vi "template-state-machine-cDAQ-AO.vi"() -> ()   [LabVIEW 2024]
uses:
  state-enum.ctl
  utils-sub-vi/csv-file-logging-util/filepath-selection.ctl
  utils-sub-vi/csv-file-logging-util/datalogging-options.ctl
  cDAQ-options.ctl
  sensor-options.ctl
  <vilib>/DAQmx/write.llb/DAQmx Write (Analog DBL 1Chan 1Samp).vi
  <vilib>/DAQmx/create/channels.llb/DAQmx Create Channel (AO-Voltage-Basic).vi
  <vilib>/DAQmx/miscellaneous.llb/DAQmx Fill In Error Info.vi
panel:
  out "Log File Open":bool
  in  "Tab Control":enum32{"Data", "Settings"}(tab)
  out "Vout":dbl
  in  "Pressure (Bar)":dbl(slide) min=0.0 max=3.0 scale=0.0..3.0
  out "Logged CSV out":string
  in  "Datalogging options":T1={"data-precision"=3, "Include Date"=FALSE, "Include Timestamp"=TRUE, "Include Milliseconds"=FALSE, "sample-rate (Hz)"=4.0, "Logging Active"=FALSE}
  in  "Log Filepath Selection":T2={"Log Filepath Source"=enum."Application Relative (Auto)", "Log File Path (Manual)"=path "C:/Users/dheard/Documents/0002-labview-projects/labview-template-state-machine/data", "Log File Folder Name"="data", "log file name"="log", "Include Date in Filename"=TRUE, "Include Time in Filename"=TRUE}
  in  "Serial Port Options":T3={"AO Channel"="cDAQ3Mod1/ao0", "AI Channel"="", "Simulate Hardware"=FALSE}
  in  "Sensor Options":T4={"Display Units"="PSI", "Zero Offset"=0.0, "Sensor Min"=0.0, "Sensor Max"=5.0, "Signal Min"=0.0, "Signal Max"=3.0, "Conversion Factor"=0.0}
  in  "save-settings":bool
  in  "load-settings":bool
  in  "Settings file":path
  out "Sample Rate (Hz)":dbl format="%-#3.3f"
  in  "Debug Mode":bool
  out "Loop Time (mS)":u32
  out "State:":T5
  out "error IO":errorcluster
  in  "stop":bool
  in  "start":bool
  in  "Exit":bool
  # "Template Logger"
  # "Conversion Factor to\nCalculate User Units from Sensor Units"
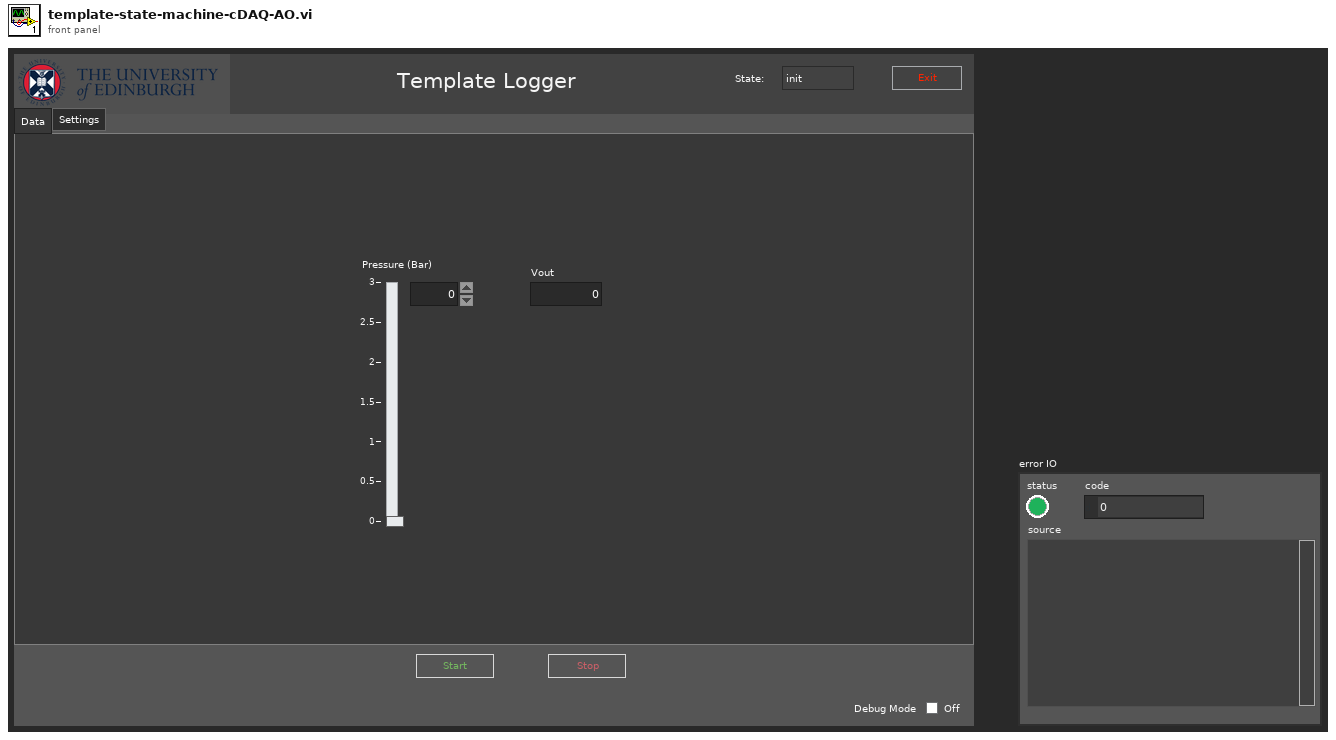
[diagram p1: front panel]
types:
  T1 = typedef "datalogging-options.ctl" = cluster{"data-precision":i32, "Include Date":bool, "Include Timestamp":bool, "Include Milliseconds":bool, "sample-rate (Hz)":dbl, "Logging Active":bool}
  T2 = typedef "filepath-selection.ctl" = cluster{"Log Filepath Source":enum16{"Application Relative (Auto)", "VI Relative (Auto)", "Complete Path (Manual)"}, "Log File Path (Manual)":path, "Log File Folder Name":string, "log file name":string, "Include Date in Filename":bool, "Include Time in Filename":bool}
  T3 = typedef "cDAQ-options.ctl" = cluster{"AO Channel":tag, "AI Channel":tag, "Simulate Hardware":bool}
  T4 = typedef "sensor-options.ctl" = cluster{"Display Units":string, "Zero Offset":dbl, "Sensor Min":dbl, "Sensor Max":dbl, "Signal Min":dbl, "Signal Max":dbl, "Conversion Factor":dbl}
  T5 = typedef "state-enum.ctl" = enum16{"init", "recall-settings", "save-settings", "wait", "start", "pre-run", "run", "stop", "shutdown", "exit"}
  T6 = enum8{"Enabled", "Disabled", "Disabled and Grayed Out"}
  T7 = enum16{"open", "replace", "create", "open or create", "replace or create", "replace or create with confirmation"}
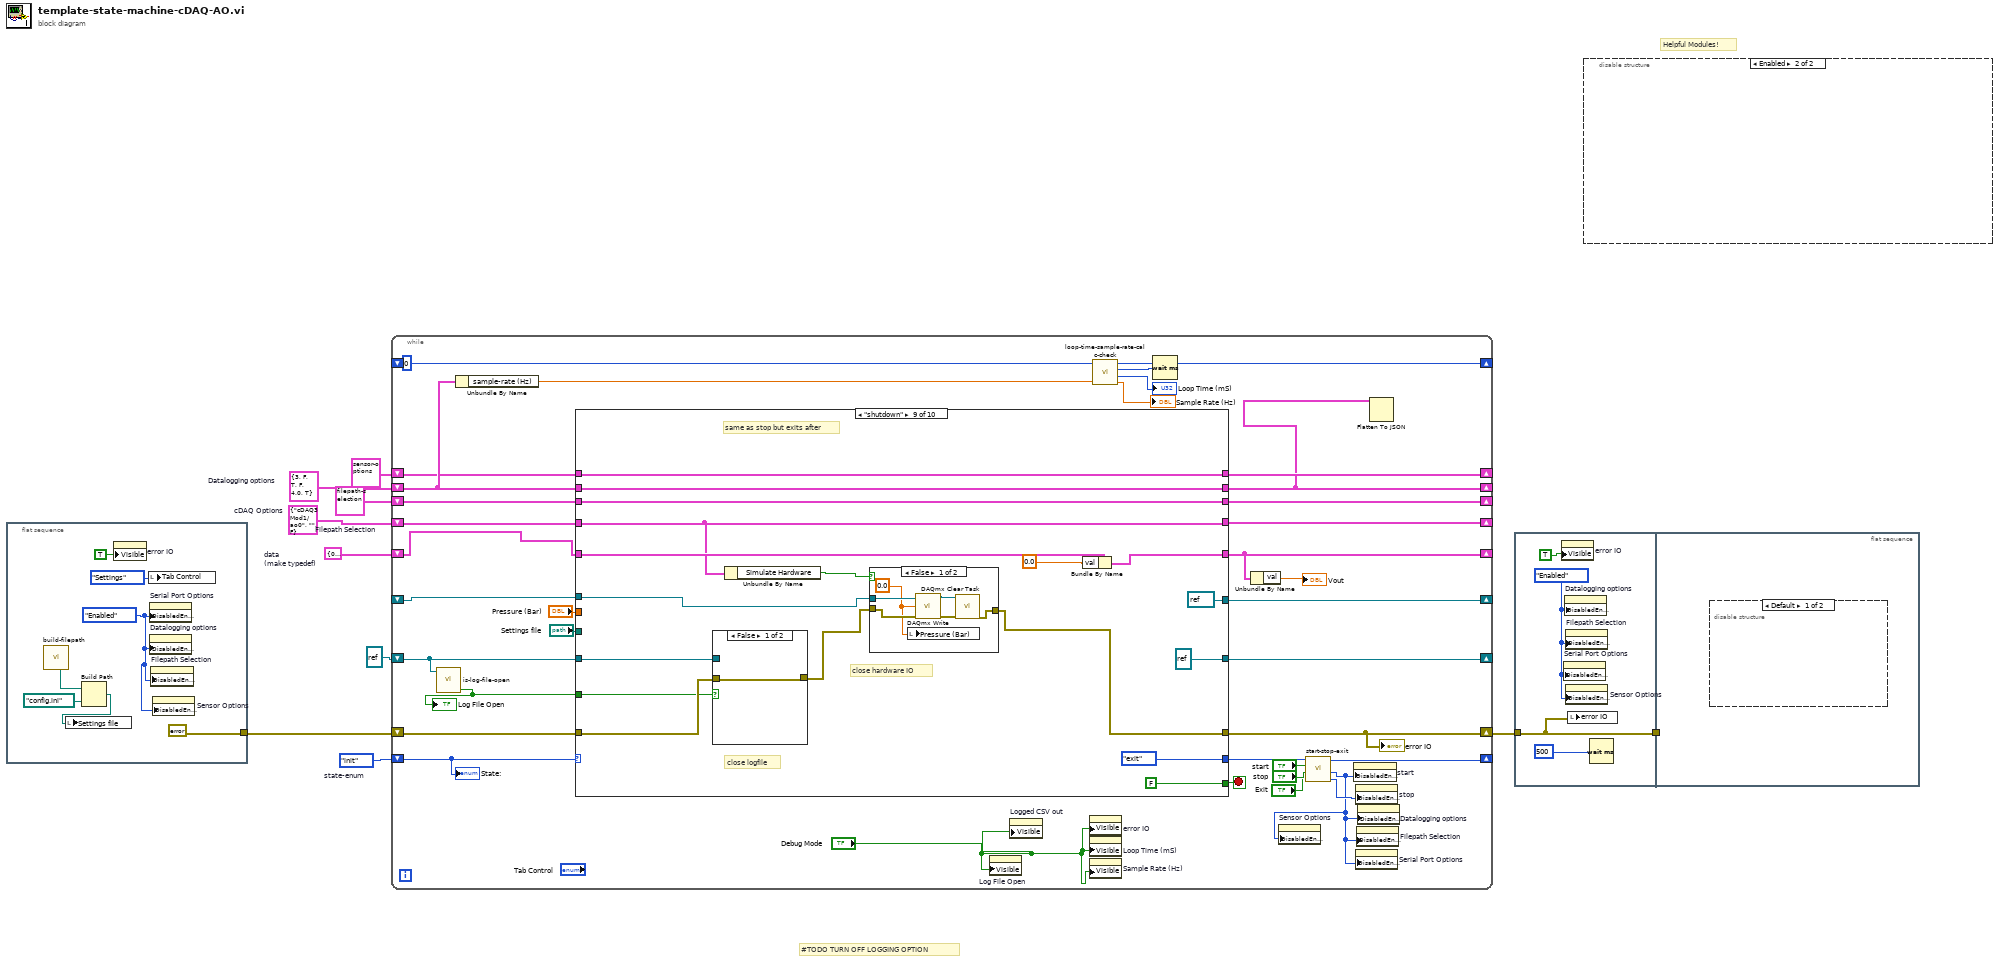
[diagram p0: block diagram]
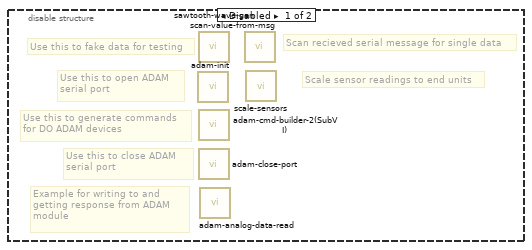
[diagram p2: hidden frame]
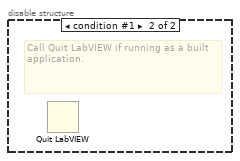
[diagram p3: hidden frame]
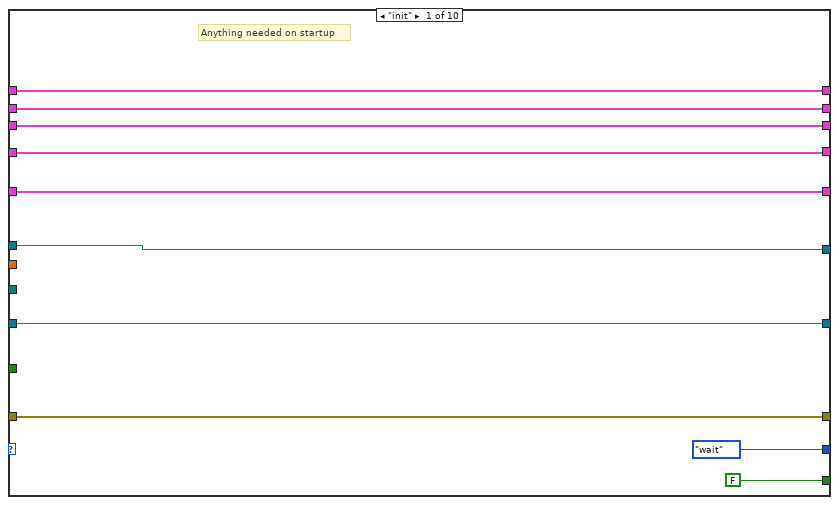
[diagram p4: hidden frame]
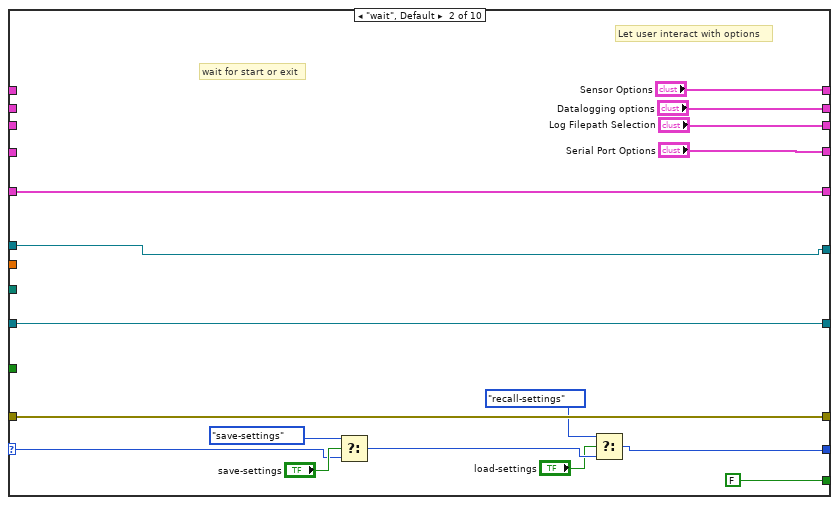
[diagram p5: hidden frame]
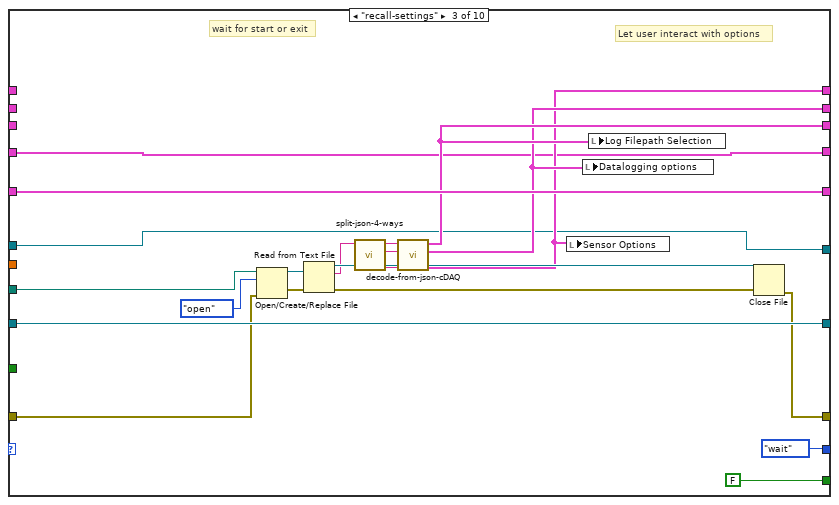
[diagram p6: hidden frame]
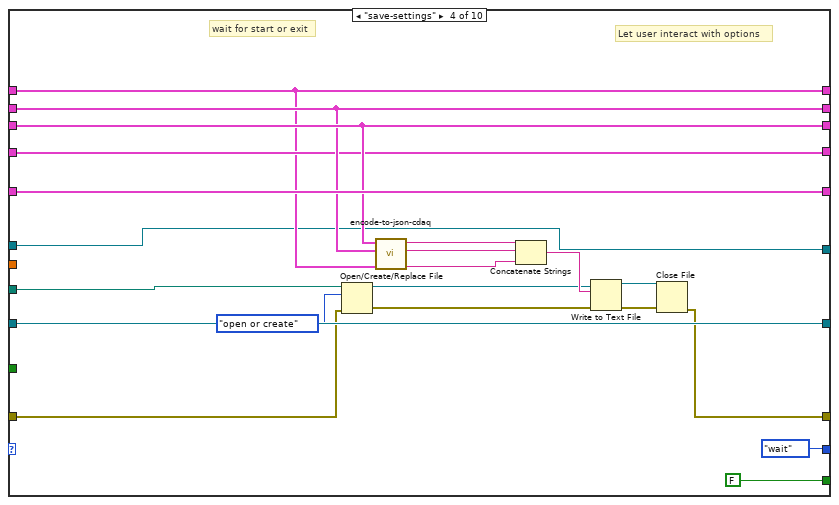
[diagram p7: hidden frame]
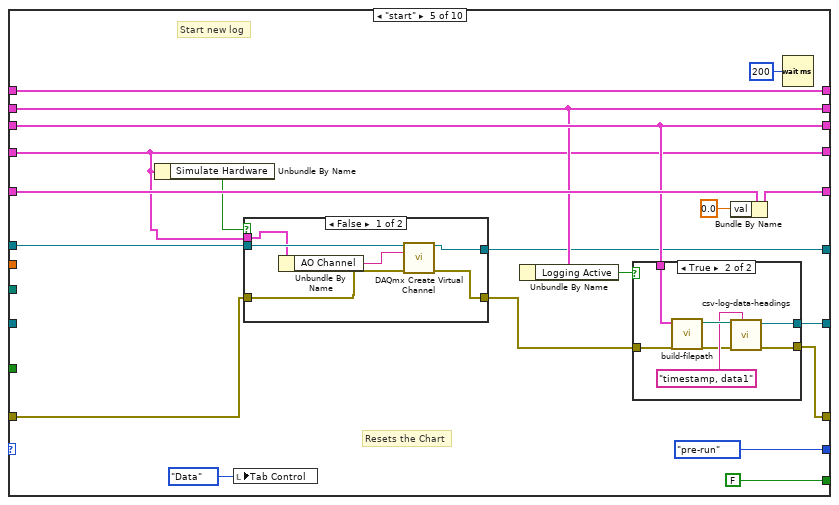
[diagram p8: hidden frame]
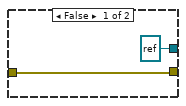
[diagram p10: hidden frame]
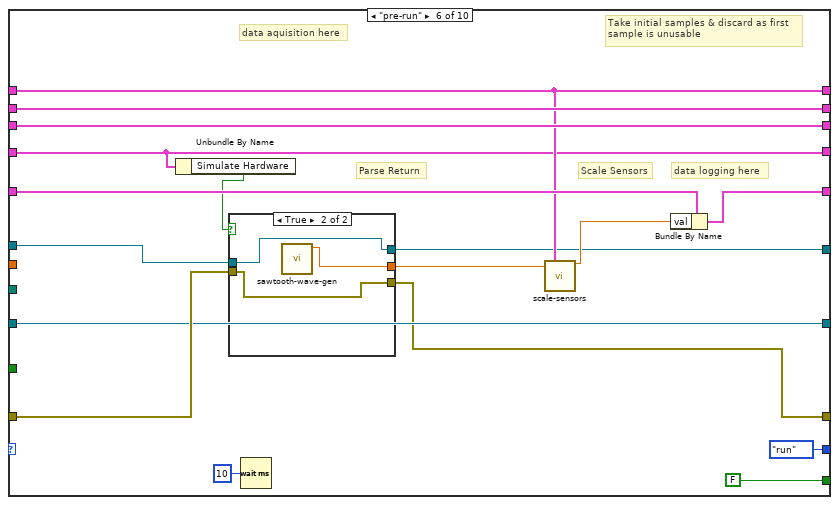
[diagram p11: hidden frame]
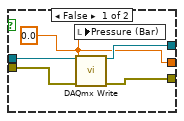
[diagram p12: hidden frame]
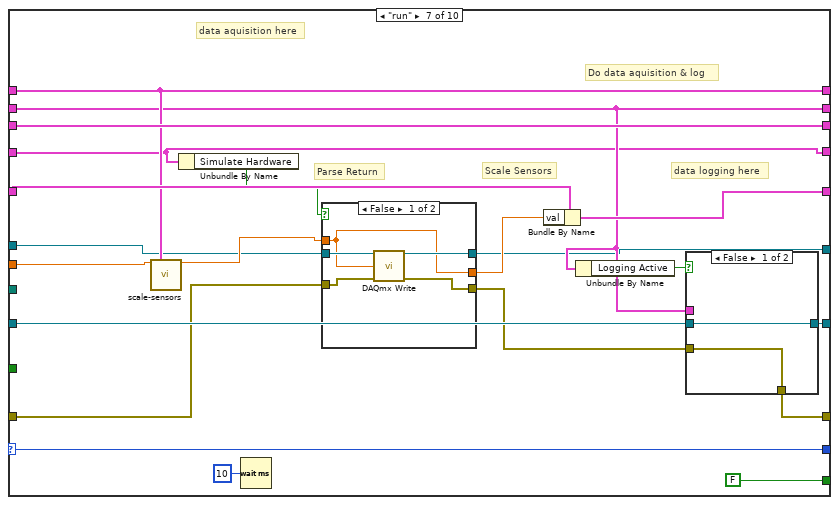
[diagram p13: hidden frame]
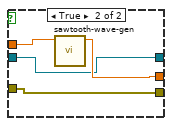
[diagram p14: hidden frame]
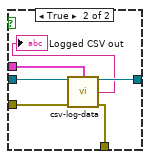
[diagram p15: hidden frame]
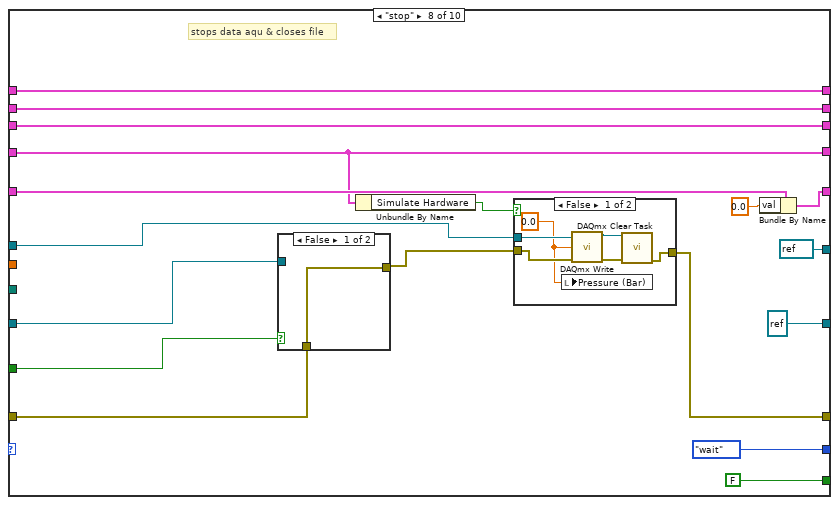
[diagram p16: hidden frame]
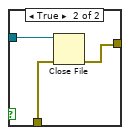
[diagram p18: hidden frame]
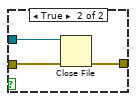
[diagram p20: hidden frame]
diagram:
  w1 = T3 {"AO Channel"="cDAQ3Mod1/ao0", "AI Channel"="", "Simulate Hardware"=FALSE}  # cDAQ Options
  w3 = T1 {"data-precision"=3, "Include Date"=FALSE, "Include Timestamp"=TRUE, "Include Milliseconds"=FALSE, "sample-rate (Hz)"=4.0, "Logging Active"=TRUE}  # Datalogging options
  w4 = T2 {"Log Filepath Source"=enum."Application Relative (Auto)", "Log File Path (Manual)"=path "C:/Users/dheard/Documents/0002-labview-projects/ammonia-absorbsion-rig/data", "Log File Folder Name"="data", "log file name"="log", "Include Date in Filename"=TRUE, "Include Time in Filename"=TRUE}  # Filepath Selection
  w8 = cluster{"val":dbl, "bool":bool, "msg":string} {"val"=0.0, "bool"=FALSE, "msg"=""}  # data (make typedef)
  w11 = state-enum."init"  # state-enum
  # "#TODO TURN OFF LOGGING OPTION"
  # "Helpful Modules!"
  n1 = flat-sequence {
    tunnel: [errorcluster {"status"=FALSE, "code"=0, "source"=""} ("error IO")] -> w7
    frame #0 {
      w15 = T6."Enabled" ("Disabled")
      n2 = call "build-filepath.vi"() -> ("Application Directory"=w14:path)  [unwired: 9 in, 2 out]
      n3 = Build Path(base path=w14, name or relative path=path "config.ini") -> (appended path=w12:path)
      n4 = local write "Settings file"(w12) -> ()
      n5 = property on="error IO" class="Clust (strict)"("Visible"=TRUE) -> ()  [unwired: 2 in, 2 out]
      n6 = local write "Tab Control"(enum32{"Data", "Settings"}."Settings" ("Tab Control")) -> ()
      n7 = property on="Serial Port Options" class="Clust (strict)"("DisabledEnum"=w15) -> ()  [unwired: 2 in, 2 out]
      n8 = property on="Datalogging options" class="Clust (strict)"("DisabledEnum"=w15) -> ()  [unwired: 2 in, 2 out]
      n9 = property on="Filepath Selection" class="Clust (strict)"("DisabledEnum"=w15) -> ()  [unwired: 2 in, 2 out]
      n10 = property on="Sensor Options" class="Clust (strict)"("DisabledEnum"=w15) -> ()  [unwired: 2 in, 2 out]
    }
  }
  n11 = while {
    shift-right: [w52] -> _
    shift-left: w11 -> [w54]
    shift-right: [w46] -> w9
    shift-left: w7 -> [w47]
    shift-right: [w20] -> _
    shift-left: w8 -> [w22]
    shift-right: [w43] -> _
    shift-left: u32 0 ("millisecond timer value") -> [w45]
    shift-right: [w39] -> _
    shift-left: w4 -> [w38]
    shift-right: [w37] -> _
    shift-left: refnum<file> refnum ("Byte Stream File out") -> [w36]
    shift-right: [w26] -> _
    shift-left: w3 -> [w34]
    shift-right: [w31] -> _
    shift-left: w1 -> [w32]
    shift-right: [w30] -> _
    shift-left: T4 {"Display Units"="units", "Zero Offset"=2.62, "Sensor Min"=0.0, "Sensor Max"=500.0, "Signal Min"=0.0, "Signal Max"=100.0, "Conversion Factor"=0.0} ("Sensor Options") -> [w28]
    shift-right: [w24] -> _
    shift-left: _ -> [w23]
    stop <- w48 stop-if-true
    n12 = call "is-log-file-open.vi"("Byte Stream File in"=w36) -> ("Log File Open"=w35:bool)  [unwired: 10 in]
    "Log File Open" <- w35
    n13 = Unbundle By Name(w34) -> ("sample-rate (Hz)"=w33:dbl)
    n14 = case shown="\"shutdown\"" w54 {
      selector: w54 -> [_ w71 _ _ _ _ w202 _ _ _]
      tunnel: [state-enum."wait" w66 state-enum."wait" state-enum."wait" state-enum."pre-run" state-enum."run" w202 state-enum."wait" state-enum."exit" state-enum."exit"] -> w53
      tunnel: [FALSE FALSE FALSE FALSE FALSE FALSE FALSE FALSE FALSE TRUE] -> w48
      tunnel: [w62 w79 w91 w104 w135 w164 w197 w227 w250 w286] -> w46
      tunnel: w47 -> [w62 w79 w95 w110 w133 w170 w196 w231 w260 w286]
      tunnel: [w61 w78 w100 w121 w138 w173 w201 w234 w263 w285] -> w20
      tunnel: w22 -> [w61 w78 w100 w121 w139 w168 w194 w236 w265 w285]
      tunnel: [w59 "Log Filepath Selection" w85 w116 w129 w172 w198 w230 w259 w283] -> w39
      tunnel: w38 -> [w59 _ _ w116 w129 w172 w198 w230 w259 w283]
      tunnel: [w60 w76 w99 w120 w136 w165 w199 refnum<file> refnum ("log file Byte Stream File out") refnum<file> refnum ("log file Byte Stream File out") w284] -> w37
      tunnel: w36 -> [w60 w76 w99 w120 _ w165 w200 w233 w262 w284]
      tunnel: [w58 "Datalogging options" w84 w115 w128 w171 w191 w229 w258 w282] -> w26
      tunnel: w34 -> [w58 _ _ w115 w128 w171 w191 w229 w258 w282]
      tunnel: w35 -> [_ _ _ _ _ _ _ w225 w257 _]
      tunnel: w32 -> [w57 _ w81 w114 w123 w161 w189 w221 w255 w281]
      tunnel: [w57 "Serial Port Options" w81 w114 w123 w161 w189 w221 w255 w281] -> w31
      tunnel: [w56 "Sensor Options" w83 w113 w131 w167 w192 w226 w256 w280] -> w30
      tunnel: w28 -> [w56 _ _ w113 w131 w167 w192 w226 w256 w280]
      tunnel: "Settings file" -> [_ _ w97 w105 _ _ _ _ _ _]
      tunnel: [w55 w65 w82 w103 w125 w158 w183 refnum<k21> refnum ("task out") refnum<k21> refnum ("task out") w279] -> w24
      tunnel: w23 -> [w55 w65 w82 w103 w124 w159 w184 w224 w252 w279]
      tunnel: "Pressure (Bar)" -> [_ _ _ _ _ _ w186 _ _ _]
      frame "init" {
        # "Anything needed on startup"
      }
      frame "wait", Default {
        # "Let user interact with options"
        # "wait for start or exit"
        n15 = Select(t=state-enum."save-settings", s="save-settings", f=w71) -> (s? t:f=w69:T5)
        n16 = Select(t=state-enum."recall-settings", s="load-settings", f=w69) -> (s? t:f=w66:T5)
      }
      frame "recall-settings" {
        # "Let user interact with options"
        # "wait for start or exit"
        n17 = Open/Create/Replace File(file path (use dialog)=w97, error in=w95, operation (0:open)=T7."open") -> (refnum out=w94:refnum<file>, error out=w93:errorcluster)  [unwired: 3 in, 1 out]
        n18 = Read from Text File(file (use dialog)=w94, error in=w93) -> (refnum out=w90:refnum<file>, text=w89:string, error out=w92:errorcluster)  [unwired: 2 in, 1 out]
        n19 = call "split-json-4-ways.vi"("json-string-in"=w89) -> ("sensor-json"=w86:string, "datalogging-json"=w87:string, "filepath-json"=w88:string)  [unwired: 7 in, 1 out]
        n20 = call "decode-from-json-cDAQ.vi"("sensor-options-json"=w86, "data-logging-json"=w87, "filepath-json"=w88) -> ("Sensor Option Recall"=w83:T4, "Datalogging Recall"=w84:T1, "Filepath Recall"=w85:T2)  [unwired: 6 in]
        n21 = local write "Sensor Options"(w83) -> ()
        n22 = local write "Datalogging options"(w84) -> ()
        n23 = local write "Log Filepath Selection"(w85) -> ()
        n24 = Close File(refnum=w90, error in=w92) -> (error out=w91:errorcluster)  [unwired: 1 out]
      }
      frame "save-settings" {
        # "Let user interact with options"
        # "wait for start or exit"
        n25 = Open/Create/Replace File(file path (use dialog)=w105, error in=w110, operation (0:open)=T7."open or create") -> (refnum out=w109:refnum<file>, error out=w108:errorcluster)  [unwired: 3 in, 1 out]
        n26 = call "encode-to-json-cdaq.vi"("Sensor Options"=w113, "Datalogging options"=w115, "Filepath Selection"=w116) -> ("sensor-options-json"=w102:string, "data-logging-json"=w117:string, "filepath-json"=w118:string)  [unwired: 6 in]
        n27 = Concatenate Strings(w118, w117, w102) -> (w112:string)
        n28 = Write to Text File(file (use dialog)=w109, text=w112, error in=w108) -> (refnum out=w107:refnum<file>, error out=w106:errorcluster)  [unwired: 1 in, 1 out]
        n29 = Close File(refnum=w107, error in=w106) -> (error out=w104:errorcluster)  [unwired: 1 out]
      }
      frame "start" {
        # "Start new log"
        # "Resets the Chart"
        n30 = Unbundle By Name(w123) -> ("Simulate Hardware"=w126:bool)
        n31 = local write "Tab Control"(enum32{"Data", "Settings"}."Data" ("Tab Control")) -> ()
        n32 = case shown="False" w126 {
          tunnel: w133 -> [w143 w149]
          tunnel: [w142 w149] -> w132
          tunnel: [w147 w148] -> w125
          tunnel: w124 -> [w146 w148]
          tunnel: w123 -> [w145 _]
          frame False {
            n33 = Unbundle By Name(w145) -> ("AO Channel"=w144:tag)
            n34 = call-poly <vilib>:"DAQmx Create Virtual Channel.vi"("task in"=w146, "physical channels"=w144, "error in"=w143) -> ("task out"=w147:refnum<k21>, "error out"=w142:errorcluster)  [unwired: 11 in]
          }
          frame True {
          }
        }
        n35 = Unbundle By Name(w128) -> ("Logging Active"=w127:bool)
        n36 = case shown="True" w127 {
          tunnel: [refnum<file> refnum ("Byte Stream File out") w155] -> w136
          tunnel: [w150 w154] -> w135
          tunnel: w132 -> [w150 w153]
          tunnel: w129 -> [_ w152]
          frame False {
          }
          frame True {
            n37 = call "build-filepath.vi"("Filepath Selection"=w152) -> ("appended path for log file"=w157:path)  [unwired: 8 in, 2 out]
            n38 = call "csv-log-data-headings.vi"("CSV Data Headings"="timestamp, data1", "error in (no error)"=w153, "Log File Path"=w157) -> ("error out"=w154:errorcluster, "Byte Stream File out"=w155:refnum<file>)  [unwired: 6 in, 1 out]
          }
        }
        n39 = Bundle By Name(cluster=w139, "val"=0.0 ("output")) -> (w138:cluster{"val":dbl, "bool":bool, "msg":string})
        n40 = Wait (ms)(milliseconds to wait=u32 200) -> ()  [unwired: 1 out]
      }
      frame "pre-run" {
        # "Take initial samples & discard as first\nsample is unusable"
        # "Scale Sensors"
        # "Parse Return"
        # "data logging here"
        # "data aquisition here"
        n41 = Unbundle By Name(w161) -> ("Simulate Hardware"=w160:bool)
        n42 = case shown="True" w160 {
          tunnel: w170 -> [w178 w181]
          tunnel: [w175 w182] -> w166
          tunnel: [w177 w181] -> w164
          tunnel: w159 -> [w179 w180]
          tunnel: [w176 w180] -> w158
          frame False {
            w175 = 0.0 ("data")
            n43 = local write "Pressure (Bar)"(w175) -> ()
            n44 = call-poly <vilib>:"DAQmx Write.vi"("task/channels in"=w179, "data"=w175, "error in"=w178) -> ("task out"=w176:refnum<k21>, "error out"=w177:errorcluster)  [unwired: 10 in, 1 out]
          }
          frame True {
            n45 = call "sawtooth-wave-gen.vi"() -> ("output"=w182:dbl)  [unwired: 11 in]
          }
        }
        n46 = Wait (ms)(milliseconds to wait=u32 10) -> ()  [unwired: 1 out]
        n47 = call "scale-sensors.vi"("Measured Value (mV)"=w166, "Sensor Options"=w167) -> ("Calculated Value (User Specified Unit)"=w162:dbl)  [unwired: 8 in, 5 out]
        n48 = Bundle By Name(cluster=w168, "val"=w162) -> (w173:cluster{"val":dbl, "bool":bool, "msg":string})
      }
      frame "run" {
        # "Scale Sensors"
        # "Parse Return"
        # "data logging here"
        # "data aquisition here"
        # "Do data aquisition & log"
        n49 = call "scale-sensors.vi"("Measured Value (mV)"=w186, "Sensor Options"=w192) -> ("Calculated Value (User Specified Unit)"=w185:dbl)  [unwired: 8 in, 5 out]
        n50 = Unbundle By Name(w189) -> ("Simulate Hardware"=w188:bool)
        n51 = Wait (ms)(milliseconds to wait=u32 10) -> ()  [unwired: 1 out]
        n52 = case shown="False" w188 {
          tunnel: w196 -> [w206 w212]
          tunnel: [w205 w212] -> w193
          tunnel: [w204 w211] -> w187
          tunnel: w185 -> [w204 w210]
          tunnel: w184 -> [w208 w209]
          tunnel: [w207 w209] -> w183
          frame False {
            n53 = call-poly <vilib>:"DAQmx Write.vi"("task/channels in"=w208, "data"=w204, "error in"=w206) -> ("task out"=w207:refnum<k21>, "error out"=w205:errorcluster)  [unwired: 10 in, 1 out]
          }
          frame True {
            n54 = call "sawtooth-wave-gen.vi"("current-val"=w210) -> ("output"=w211:dbl)  [unwired: 10 in]
          }
        }
        n55 = Bundle By Name(cluster=w194, "val"=w187) -> (w201:cluster{"val":dbl, "bool":bool, "msg":string})
        n56 = Unbundle By Name(w191) -> ("Logging Active"=w190:bool)
        n57 = case shown="False" w190 {
          tunnel: w200 -> [w214 w220]
          tunnel: [w214 w219] -> w199
          tunnel: [w213 w217] -> w197
          tunnel: w191 -> [_ w216]
          tunnel: w193 -> [w213 w215]
          frame False {
          }
          frame True {
            n58 = call "csv-log-data.vi"("log file Byte Stream File in"=w220, "Datalogging options"=w216, "error in (no error)"=w215) -> ("log file Byte Stream File out"=w219:refnum<file>, "Logged CSV out"=→"Logged CSV out":string, "error out"=w217:errorcluster)  [unwired: 8 in, 2 out]
          }
        }
      }
      frame "stop" {
        # "stops data aqu & closes file"
        n59 = case shown="False" w225 {
          tunnel: w233 -> [_ w249]
          tunnel: w231 -> [w246 w248]
          tunnel: [w246 w247] -> w228
          frame False {
          }
          frame True {
            n60 = Close File(refnum=w249, error in=w248) -> (error out=w247:errorcluster)  [unwired: 1 out]
          }
        }
        n61 = Unbundle By Name(w221) -> ("Simulate Hardware"=w222:bool)
        n62 = case shown="False" w222 {
          tunnel: w228 -> [w241 w245]
          tunnel: [w244 w245] -> w227
          tunnel: w224 -> [w243 _]
          frame False {
            w239 = 0.0 ("data")
            n63 = local write "Pressure (Bar)"(w239) -> ()
            n64 = call-poly <vilib>:"DAQmx Write.vi"("task/channels in"=w243, "data"=w239, "error in"=w241) -> ("task out"=w242:refnum<k21>, "error out"=w240:errorcluster)  [unwired: 10 in, 1 out]
            n65 = call <vilib>:"DAQmx Clear Task.vi"("task in"=w242, "error in"=w240) -> ("error out"=w244:errorcluster)  [unwired: 13 in]
          }
          frame True {
          }
        }
        n66 = Bundle By Name(cluster=w236, "val"=0.0 ("output")) -> (w234:cluster{"val":dbl, "bool":bool, "msg":string})
      }
      frame "shutdown" {
        # "close hardware IO"
        # "close logfile"
        # "same as stop but exits after"
        n67 = case shown="False" w257 {
          tunnel: w262 -> [_ w278]
          tunnel: w260 -> [w275 w277]
          tunnel: [w275 w276] -> w251
          frame False {
          }
          frame True {
            n68 = Close File(refnum=w278, error in=w277) -> (error out=w276:errorcluster)  [unwired: 1 out]
          }
        }
        n69 = Unbundle By Name(w255) -> ("Simulate Hardware"=w253:bool)
        n70 = case shown="False" w253 {
          tunnel: w251 -> [w270 w274]
          tunnel: [w273 w274] -> w250
          tunnel: w252 -> [w272 _]
          frame False {
            w268 = 0.0 ("data")
            n71 = local write "Pressure (Bar)"(w268) -> ()
            n72 = call-poly <vilib>:"DAQmx Write.vi"("task/channels in"=w272, "data"=w268, "error in"=w270) -> ("task out"=w271:refnum<k21>, "error out"=w269:errorcluster)  [unwired: 10 in, 1 out]
            n73 = call <vilib>:"DAQmx Clear Task.vi"("task in"=w271, "error in"=w269) -> ("error out"=w273:errorcluster)  [unwired: 13 in]
          }
          frame True {
          }
        }
        n74 = Bundle By Name(cluster=w265, "val"=0.0 ("output")) -> (w263:cluster{"val":dbl, "bool":bool, "msg":string})
      }
      frame "exit" {
        # "Exit safely"
      }
    }
    "error IO" <- w46
    n75 = property on="Log File Open" class="Bool (strict)"("Visible"="Debug Mode") -> ()  [unwired: 2 in, 2 out]
    n76 = property on="Logged CSV out" class="Str"("Visible"="Debug Mode") -> ()  [unwired: 2 in, 2 out]
    n77 = property on="error IO" class="Clust (strict)"("Visible"="Debug Mode") -> ()  [unwired: 2 in, 2 out]
    n78 = property on="Loop Time (mS)" class="DigNum (strict)"("Visible"="Debug Mode") -> ()  [unwired: 2 in, 2 out]
    n79 = property on="Sample Rate (Hz)" class="DigNum (strict)"("Visible"="Debug Mode") -> ()  [unwired: 2 in, 2 out]
    n80 = call "loop-time-sample-rate-calc-check.vi"("sample-rate-Hz"=w33, "millisecond timer value in"=w45) -> ("Loop Hz"=→"Sample Rate (Hz)":dbl, "Loop Time (mS)"=→"Loop Time (mS)":u32, "sample-rate-delay-mS"=w40:u32, "millisecond timer value out"=w43:u32)  [unwired: 6 in]
    n81 = Wait (ms)(milliseconds to wait=w40) -> ()  [unwired: 1 out]
    n82 = Unbundle By Name(w20) -> ("val"=→"Vout":dbl)
    n83 = call "start-stop-exit.vi"("Exit"="Exit", "stop"="stop", "start"="start", "current-state"=w53) -> ("stop-enable"=w44:T6, "start-enable"=w29:T6, "new-state"=w52:T5)  [unwired: 5 in]
    n84 = property on="Sensor Options" class="Clust (strict)"("DisabledEnum"=w29) -> ()  [unwired: 2 in, 2 out]
    n85 = property on="start" class="Bool"("DisabledEnum"=w29) -> ()  [unwired: 2 in, 2 out]
    n86 = property on="stop" class="Bool"("DisabledEnum"=w44) -> ()  [unwired: 2 in, 2 out]
    n87 = property on="Serial Port Options" class="Clust (strict)"("DisabledEnum"=w29) -> ()  [unwired: 2 in, 2 out]
    n88 = property on="Filepath Selection" class="Clust (strict)"("DisabledEnum"=w29) -> ()  [unwired: 2 in, 2 out]
    n89 = property on="Datalogging options" class="Clust (strict)"("DisabledEnum"=w29) -> ()  [unwired: 2 in, 2 out]
    n90 = Flatten To JSON(anything=w26) -> ()  [unwired: 2 in, 2 out]
    "State:" <- w54
  }
  n91 = flat-sequence {
    tunnel: [w290] -> w10
    tunnel: w9 -> [w290]
    tunnel: w10 -> [_]
    frame #0 {
      w289 = T6."Enabled" ("Disabled")
      n92 = property on="error IO" class="Clust (strict)"("Visible"=TRUE) -> ()  [unwired: 2 in, 2 out]
      n93 = property on="Serial Port Options" class="Clust (strict)"("DisabledEnum"=w289) -> ()  [unwired: 2 in, 2 out]
      n94 = property on="Datalogging options" class="Clust (strict)"("DisabledEnum"=w289) -> ()  [unwired: 2 in, 2 out]
      n95 = property on="Filepath Selection" class="Clust (strict)"("DisabledEnum"=w289) -> ()  [unwired: 2 in, 2 out]
      n96 = property on="Sensor Options" class="Clust (strict)"("DisabledEnum"=w289) -> ()  [unwired: 2 in, 2 out]
      n97 = local write "error IO"(w290) -> ()
      n98 = Wait (ms)(milliseconds to wait=u32 500) -> ()  [unwired: 1 out]
    }
    frame #1 {
      n99 = disable-structure "Conditional Disable Structure" shown="Default" {
        frame condition #0 (active) {
        }
        frame condition #1 {
          # "Call Quit LabVIEW if running as a built application."
          n100 = Quit LabVIEW() -> ()  [unwired: 1 in]
        }
      }
    }
  }
  n101 = disable-structure shown="Enabled" {
    frame Disabled {
      # "Scale sensor readings to end units"
      # "Scan recieved serial message for single data"
      # "Example for writing to and\ngetting response from ADAM\nmodule"
      # "Use this to open ADAM\nserial port"
      # "Use this to close ADAM \nserial port"
      # "Use this to generate commands\nfor DO ADAM devices"
      # "Use this to fake data for testing"
      n102 = call "adam-init.vi"() -> ()  [unwired: 10 in, 2 out]
      n103 = call "sawtooth-wave-gen.vi"() -> ()  [unwired: 11 in, 1 out]
      n104 = call "adam-cmd-builder-2(SubVI).vi"() -> ()  [unwired: 6 in, 6 out]
      n105 = call "adam-close-port.vi"() -> ()  [unwired: 11 in, 1 out]
      n106 = call "adam-analog-data-read.vi"() -> ()  [unwired: 7 in, 5 out]
      n107 = call "scan-value-from-msg.vi"() -> ()  [unwired: 9 in, 3 out]
      n108 = call "scale-sensors.vi"() -> ()  [unwired: 10 in, 6 out]
    }
    frame Enabled {
    }
  }
